vi "Set Color.vi"(8 "error in (no error)":errorcluster, 10 "Color Message.lvclass":refnum<class "Color Message.lvclass">, 11 "Setting View in":refnum<class "Setting View.lvclass">) -> (0 "error out":errorcluster, 3 "Setting View out":refnum<class "Setting View.lvclass">)   [LabVIEW 2020, in "[V]Setting View.lvlib" / "Setting View.lvclass"]
uses:
  Setting View.lvclass
  Color Interface/Color/Color Message.lvclass
  Color Interface/Color/Color Message.lvclass/Color Message.ctl
  Setting View.lvclass/Setting View.ctl
  Depden On/Abstruct View/Abstruct View/Abstruct View.lvclass/Abstruct View.ctl
  Color Interface/Color/Accessors/Read BG Color.vi
  Color Interface/Color/Accessors/Read Fornt Color.vi
  Depden On/Abstruct View/Abstruct View/Data Accessors/Read Core VI.vi
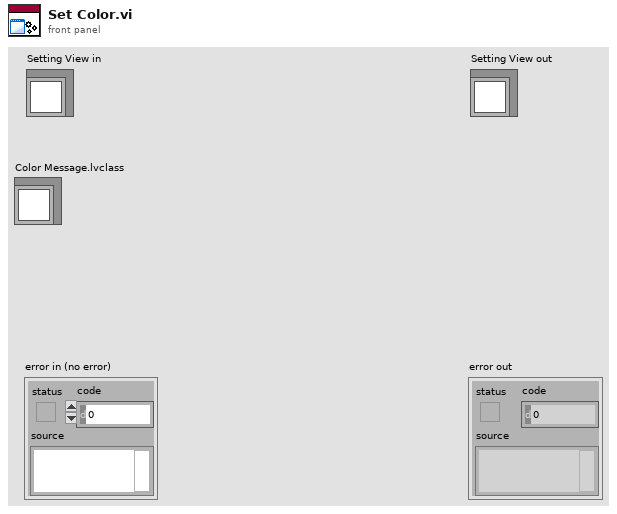
[diagram p1: front panel]
types:
  T1 = cluster{"Color Box 2":u32, "Accessors:Fornt Color":u32}
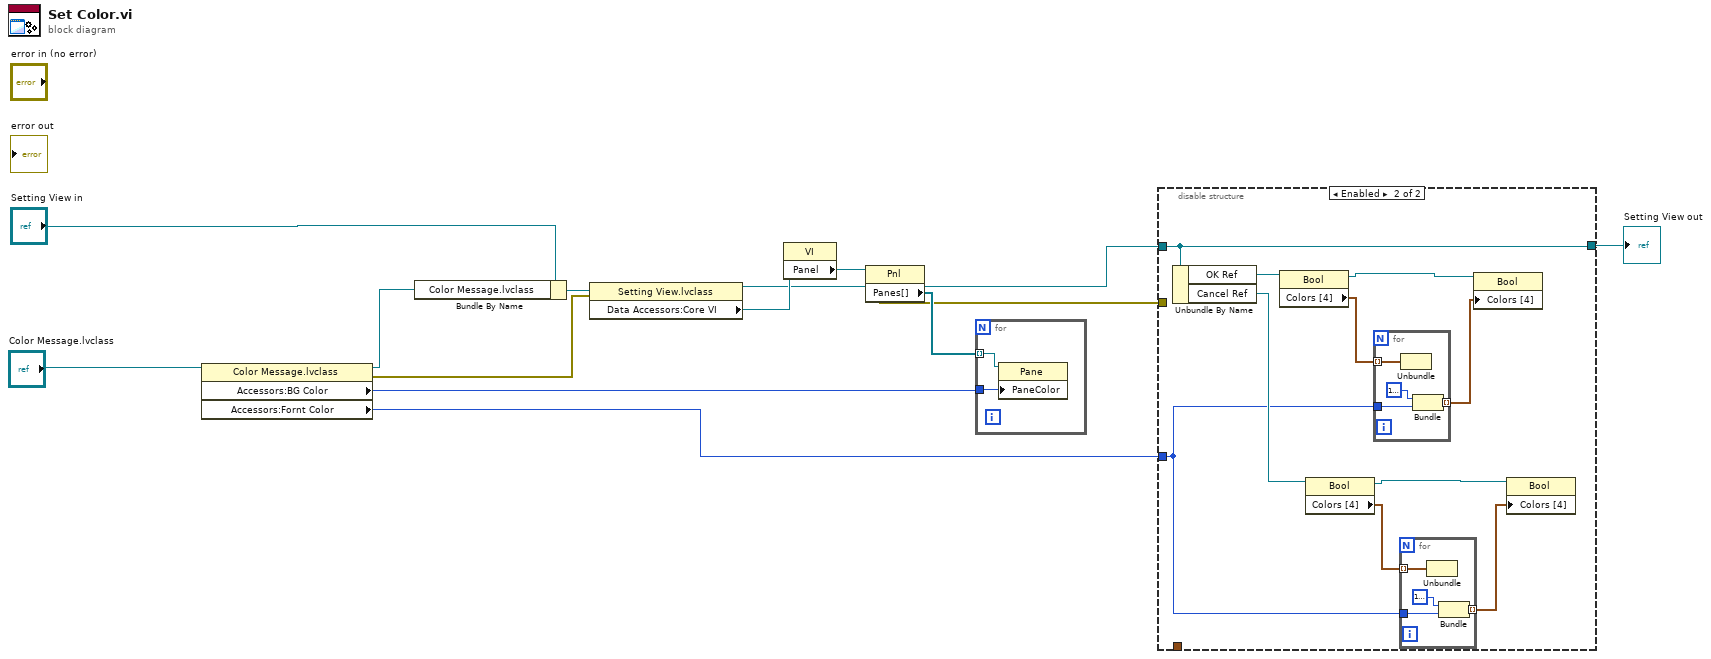
[diagram p0: block diagram]
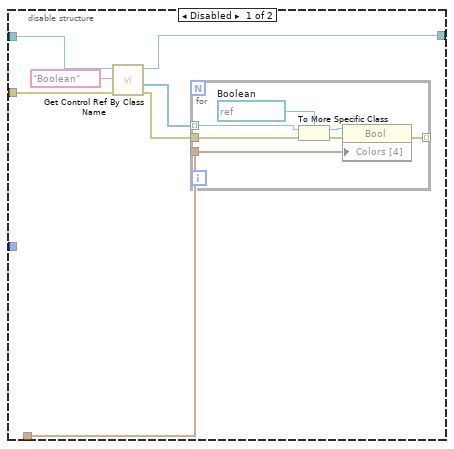
[diagram p2: hidden frame]
diagram:
  n1 = property class="Color Message.lvclass"(reference="Color Message.lvclass") -> (reference out=w1:refnum<class "Color Message.lvclass">, error out=w2:errorcluster, "Accessors:BG Color"=w7:u32, "Accessors:Fornt Color"=w6:u32)  [unwired: 1 in]
  n2 = Bundle By Name(cluster="Setting View in", "Color Message.lvclass"=w1) -> (w3:refnum<class "Setting View.lvclass">)
  n3 = property class="Setting View.lvclass"(reference=w3, error in=w2) -> (reference out=w11:refnum<class "Setting View.lvclass">, "Data Accessors:Core VI"=w13:refnum<vi>)  [unwired: 1 out]
  n4 = property class="VI"(reference=w13) -> ("Panel"=w12:refnum<vi>)  [unwired: 1 in, 2 out]
  n5 = property class="Pnl"(reference=w12) -> (error out=w8:errorcluster, "Panes[]"=w9:refnum<vi>[])  [unwired: 1 in, 1 out]
  n6 = for {
    tunnel: w9 -> [w15] mode=indexing
    tunnel: w7 -> [w14]
    n7 = property class="Pane"(reference=w15, "PaneColor"=w14) -> ()  [unwired: 1 in, 2 out]
  }
  n8 = disable-structure shown="Enabled" {
    disable-tunnel: w11 -> [w22 w39]
    disable-tunnel: [w21 w39] -> w10
    disable-tunnel: w8 -> [w19 _]
    disable-tunnel: _ -> [w17 _]
    disable-tunnel: w6 -> [_ w30]
    frame Disabled {
      n9 = call "Get Control Ref By Class Name.vi"("error in (no error)"=w19, "Control Class"="Boolean", "Setting View in"=w22) -> ("error out"=w16:errorcluster, "refs"=w18:refnum<vi>[], "Setting View out"=w21:refnum<class "Setting View.lvclass">)  [unwired: 6 in]
      n10 = for {
        tunnel: w18 -> [w29] mode=indexing
        tunnel: w17 -> [w25]
        tunnel: w16 -> [w24]
        tunnel: [w23] -> _ mode=indexing
        w28 = refnum<vi> refnum  # Boolean
        n11 = To More Specific Class(target class=w28, reference=w29, error in=w24) -> (specific class reference=w27:refnum<vi>, error out=w26:errorcluster)
        n12 = property class="Bool"(reference=w27, error in=w26, "Colors [4]"=w25) -> (error out=w23:errorcluster)  [unwired: 1 out]
      }
    }
    frame Enabled {
      n13 = Unbundle By Name(w39) -> ("OK Ref"=w38:refnum<vi>, "Cancel Ref"=w31:refnum<vi>)
      n14 = property class="Bool"(reference=w38) -> (reference out=w37:refnum<vi>, "Colors [4]"=w36:cluster{u32, u32}[])  [unwired: 1 in, 1 out]
      n15 = property class="Bool"(reference=w31) -> (reference out=w32:refnum<vi>, "Colors [4]"=w33:cluster{u32, u32}[])  [unwired: 1 in, 1 out]
      n16 = for {
        tunnel: w36 -> [w47] mode=indexing
        tunnel: w30 -> [w45]
        tunnel: [w46] -> w35 mode=indexing
        n17 = Unbundle(w47) -> ()  [unwired: 2 out]
        n18 = Bundle("Color Box 2"=u32 16777216, "Accessors:Fornt Color"=w45) -> (w46:T1)  [unwired: 1 in]
      }
      n19 = for {
        tunnel: w33 -> [w43] mode=indexing
        tunnel: w30 -> [w41]
        tunnel: [w42] -> w34 mode=indexing
        n20 = Unbundle(w43) -> ()  [unwired: 2 out]
        n21 = Bundle("Color Box 2"=u32 16777216, "Accessors:Fornt Color"=w41) -> (w42:T1)  [unwired: 1 in]
      }
      n22 = property class="Bool"(reference=w37, "Colors [4]"=w35) -> ()  [unwired: 1 in, 2 out]
      n23 = property class="Bool"(reference=w32, "Colors [4]"=w34) -> ()  [unwired: 1 in, 2 out]
    }
  }
  "Setting View out" <- w10
